vi "Plot axes grid colors.vi"(8 "error in (no error)":errorcluster, 10 "Scale reference":refnum<vi>, 11 "Meta LUT":refnum<data-value>) -> (0 "error out":errorcluster, 2 "Scale reference":refnum<vi>, 3 "Meta LUT":refnum<data-value>)   [LabVIEW 2021, in "RocketPlot.lvlib"]
uses:
  RocketPlot.lvlib
  Plot scale refnum to LUT name.vi
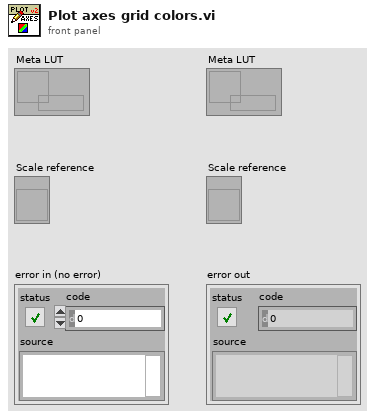
[diagram p1: front panel]
types:
  T1 = typedef "RocketPlot.lvlib/Plot scale meta JSON.ctl" = cluster{"Type":T2, "Grid Colors:Major Color":u32, "Grid Colors:Minor Color":u32, "Style":u8, "Tick Colors:Tick Color":u32, "Tick Colors:Minor Tick Color":u32, "Format String":string, "State":T3, "AxisFocus":refnum<vi>}
  T2 = typedef "RocketPlot.lvlib/Plot axis.ctl" = enum16{"x axis", "left axis", "right axis"}
  T3 = typedef "RocketPlot.lvlib/Plot scale meta state.ctl" = cluster{"Visible":bool, "Focus":bool, "Multi-Y":bool}
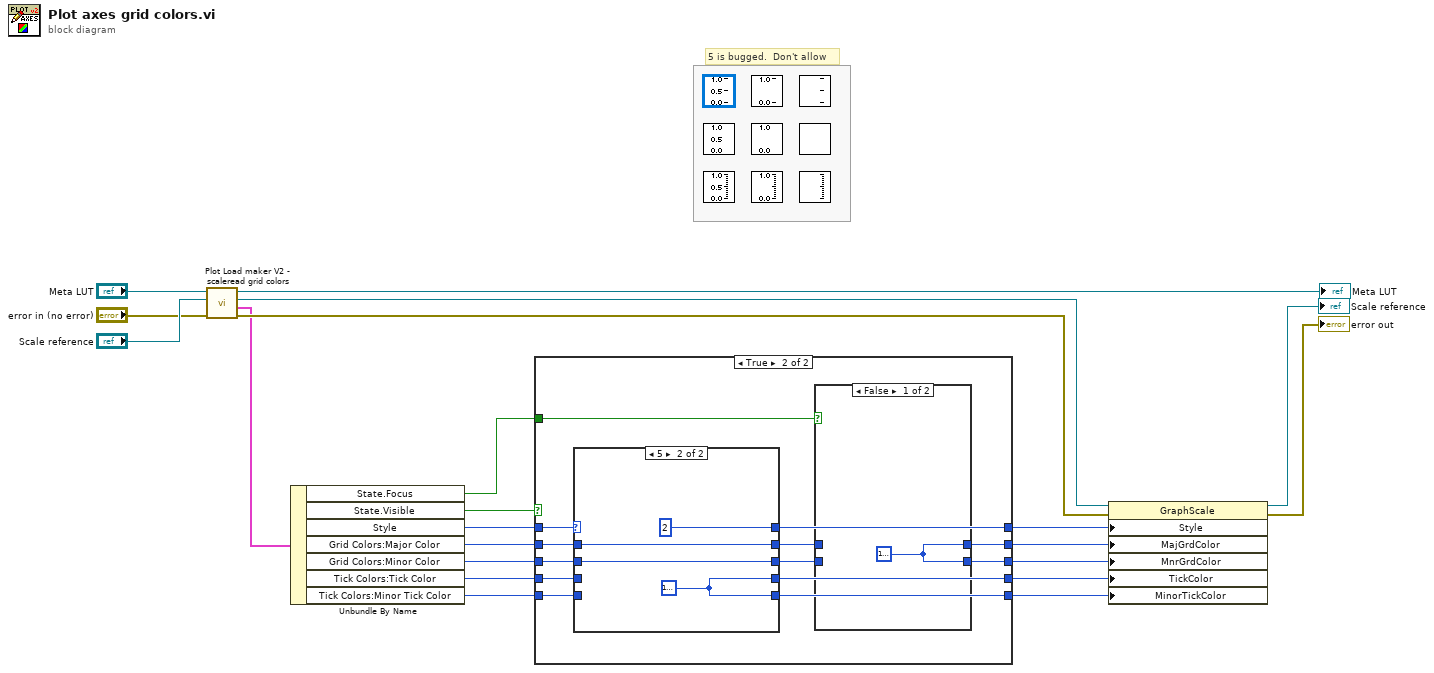
[diagram p0: block diagram]
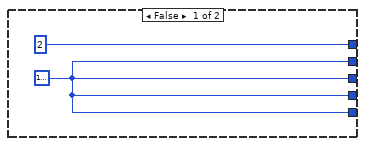
[diagram p2: hidden frame]
diagram:
  # "5 is bugged.  Don't allow"
  n1 = call "Plot Load maker V2 - scaleread grid colors.vi"("error in (no error)"="error in (no error)", "Scale reference"="Scale reference", "Meta LUT"="Meta LUT") -> ("error out"=w19:errorcluster, "Scale LUT meta"=w17:T1, "Scale reference"=w20:refnum<vi>, "Meta LUT"=→"Meta LUT":refnum<data-value>)  [unwired: 5 in]
  n2 = Unbundle By Name(w17) -> ("State.Focus"=w2:bool, "State.Visible"=w16:bool, "Style"=w12:u8, "Grid Colors:Major Color"=w11:u32, "Grid Colors:Minor Color"=w10:u32, "Tick Colors:Tick Color"=w6:u32, "Tick Colors:Minor Tick Color"=w5:u32)
  n3 = case shown="True" w16 {
    tunnel: [w22 w30] -> w15
    tunnel: [w22 w28] -> w14
    tunnel: [u8 2 ("invisible scale Style") w26] -> w13
    tunnel: w12 -> [_ w36]
    tunnel: w11 -> [_ w35]
    tunnel: w10 -> [_ w34]
    tunnel: w6 -> [_ w33]
    tunnel: w5 -> [_ w32]
    tunnel: [w22 w25] -> w4
    tunnel: [w22 w24] -> w3
    tunnel: w2 -> [_ w31]
    frame False {
      w22 = u32 16777216
    }
    frame True {
      n4 = case shown="5" w36 {
        selector: w36 -> [w44 _]
        tunnel: [w44 u8 2 ("invisible scale Style")] -> w26
        tunnel: [w43 w47] -> w29
        tunnel: [w42 w46] -> w27
        tunnel: w35 -> [w43 w47]
        tunnel: w34 -> [w42 w46]
        tunnel: w33 -> [w41 _]
        tunnel: [w41 w45] -> w25
        tunnel: [w40 w45] -> w24
        tunnel: w32 -> [w40 _]
        frame Default {
        }
        frame 5 {
          w45 = u32 16777216
        }
      }
      n5 = case shown="False" w31 {
        tunnel: [w37 w39] -> w30
        tunnel: w29 -> [_ w39]
        tunnel: [w37 w38] -> w28
        tunnel: w27 -> [_ w38]
        frame False {
          w37 = u32 16777216
        }
        frame True {
        }
      }
    }
  }
  n6 = property class="GraphScale"(reference=w20, error in=w19, "Style"=w13, "MajGrdColor"=w15, "MnrGrdColor"=w14, "TickColor"=w4, "MinorTickColor"=w3) -> (reference out=→"Scale reference":refnum<vi>, error out=→"error out":errorcluster)
